vi "meas_voltmetr_with_scanner.vi"(8 "error in (no error)":errorcluster, 9 "Range":dbl=-1.0, 10 "Function":T1, 11 "output cluster in":T2) -> (0 "error out":errorcluster, 2 "value":dbl, 3 "output cluster out":T2)   [LabVIEW 2017]
uses:
  controls/app_data.ctl
  controls/instruments.ctl
  Unicorn Labview Library/Control/unicorn_Param.ctl
  Unicorn Labview Library/Control/unicorn_conn.ctl
  Unicorn Labview Library/Control/unicorn_JSON.ctl
  Unicorn Labview Library/Control/unicorn_ParamInt.ctl
  Unicorn Labview Library/Control/unicorn_Telemetry.ctl
  Unicorn Labview Library/Control/unicorn_Table.ctl
  Unicorn Labview Library/Control/unicorn_ParamFloat.ctl
  <instrlib>/PICOTEST M352XA/Public/Controls/Function.ctl
  Unicorn Labview Library/Unicorn Library.lvlib
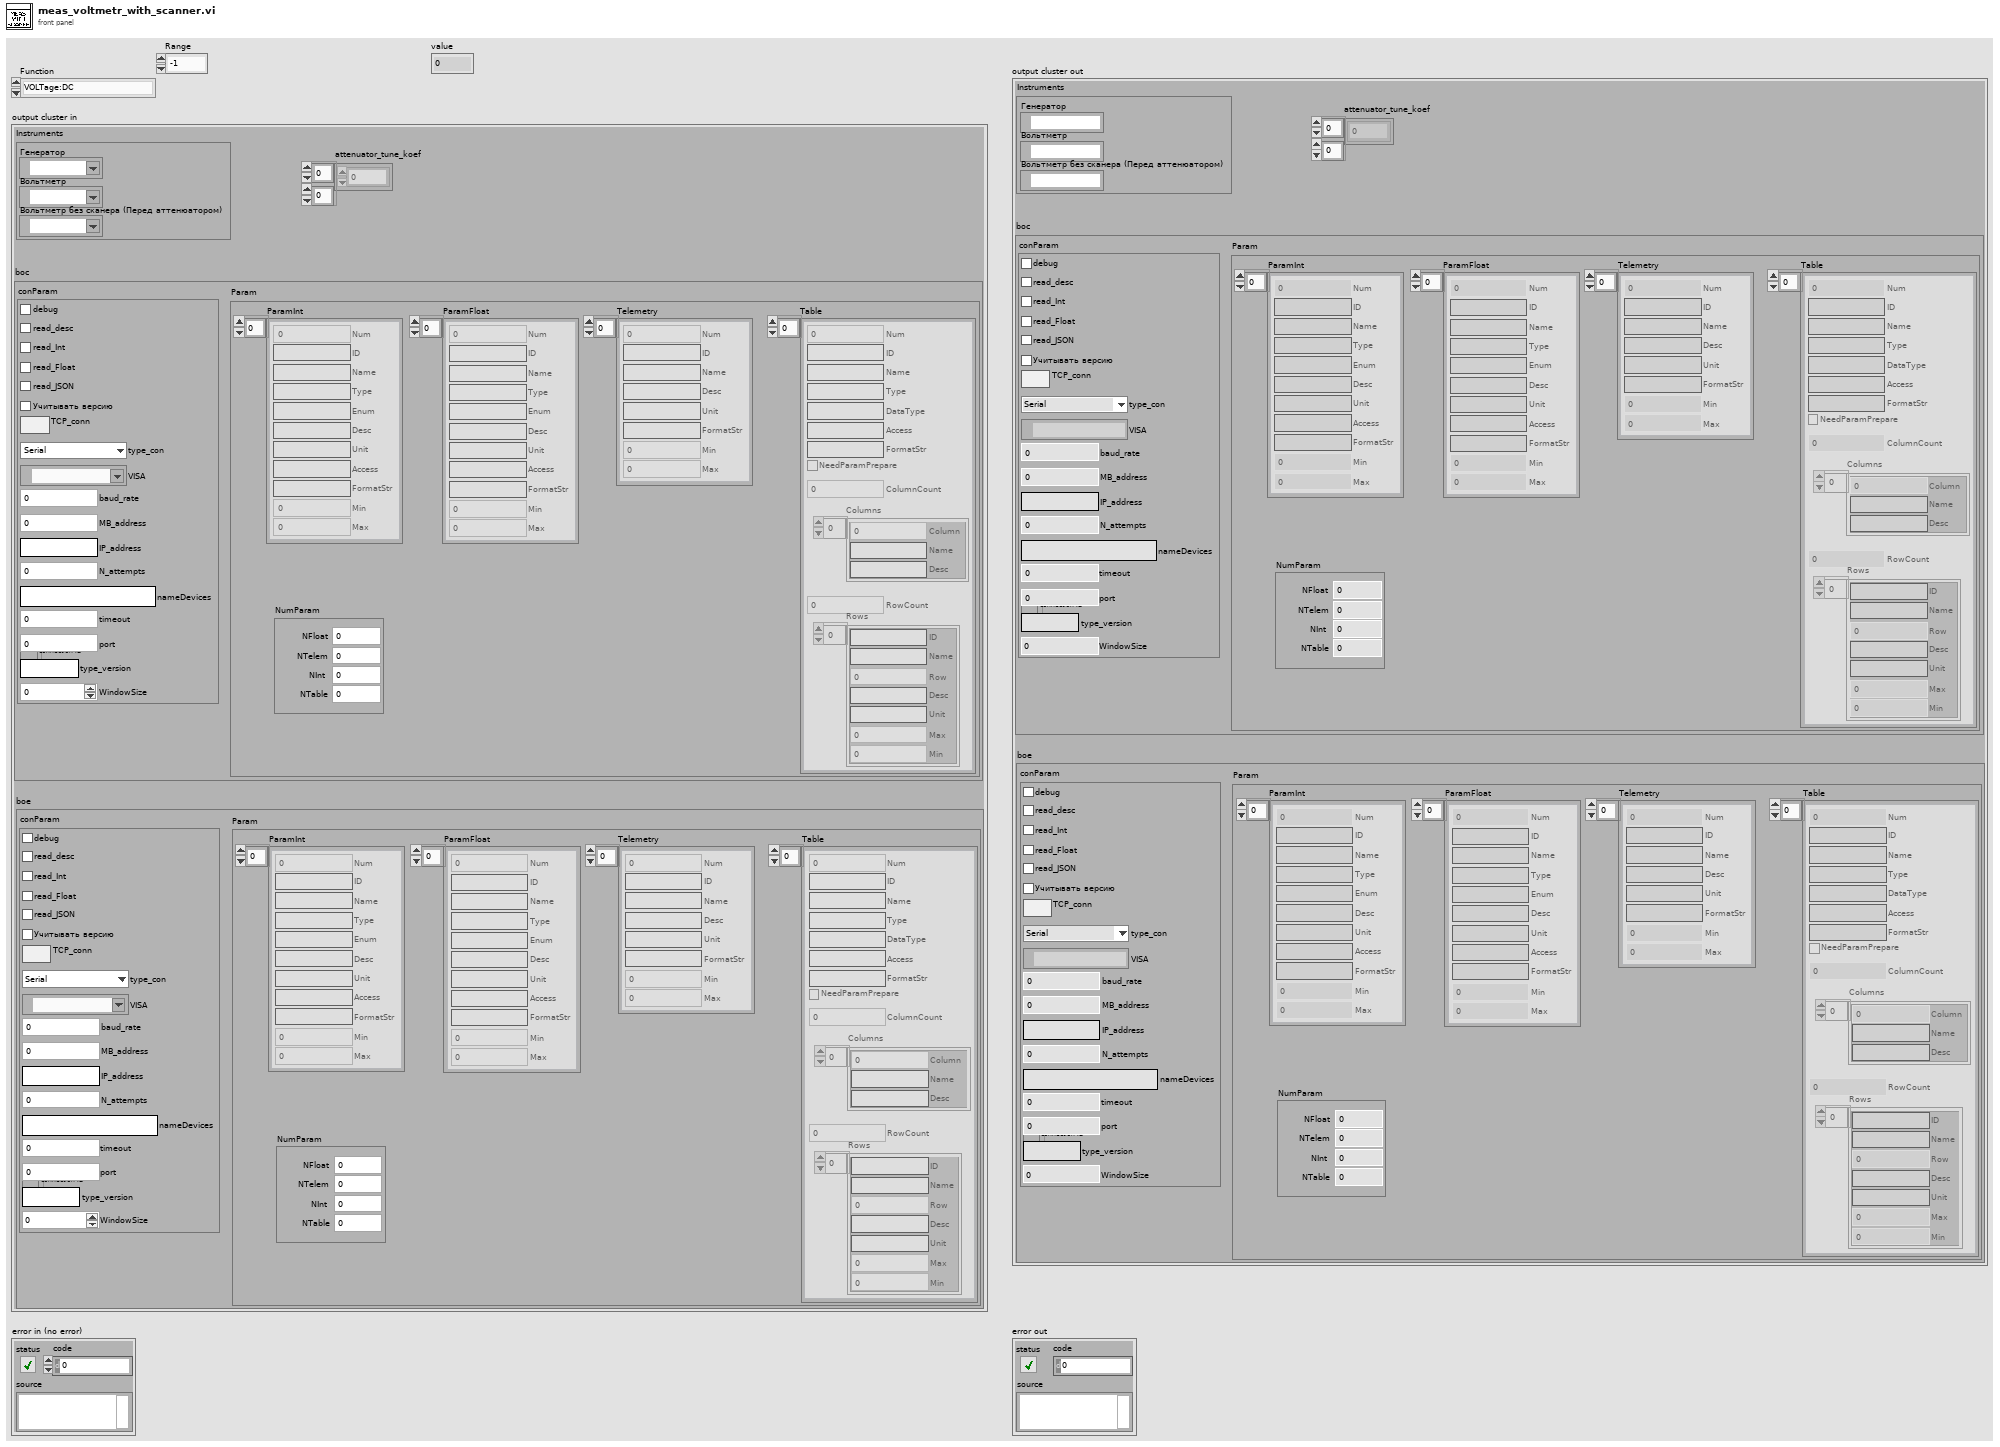
[diagram p1: front panel]
types:
  T1 = typedef "Function.ctl" = enum16{"VOLTage:DC", "VOLTage:DC:RATio", "VOLTage:AC", "CURRent:DC", "CURRent:AC", "RESistance", "FRESistance", "FREQuency", "PERiod", "FREQuency:CURRent", "PERiod:CURRent", "CAPacitance", "CONTinuity", "DIODe", "TCOuple", "TEMPerature"}
  T2 = typedef "app_data.ctl" = cluster{"Instruments":T3, "boc":T4, "boe":T4, "attenuator_tune_koef":dbl[][]}
  T3 = typedef "instruments.ctl" = cluster{"generator":refnum<visa-resource-name>, "voltment_with_scaner":refnum<visa-resource-name>, "voltment_without_scaner":refnum<visa-resource-name>}
  T4 = typedef "Unicorn Library.lvlib/unicorn_Param.ctl" = cluster{"conParam":T5, "Param":T6}
  T5 = typedef "Unicorn Library.lvlib/unicorn_conn.ctl" = cluster{"ReadIntParam":bool, "ReadDescrParam":bool, "ReadFloatParam":bool, "debug":bool, "ReadJSON":bool, "IP_address":string, "N_attempts":i32, "type_con":enum16{"Serial", "TCP"}, "MB_address":i32, "VISA":refnum<visa-resource-name>, "connection ID":refnum<k5>, "nameDevices":string, "timeout":i32, "port":u16, "type_version":string, "baud_rate":u32, "VersionControl":bool, "TCP_conn":bool, "WindowSize":i32}
  T6 = typedef "Unicorn Library.lvlib/unicorn_JSON.ctl" = cluster{"NumParam":cluster{"NTelem":i32, "NInt":i32, "NFloat":i32, "NTable":i32}, "ParamInt":T7, "Telemetry":T8, "Table":T9, "ParamFloat":T10}
  T7 = typedef "Unicorn Library.lvlib/unicorn_ParamInt.ctl" = cluster{"ID":string, "Num":i32, "Name":string, "Type":string, "Enum":string, "Desc":string, "Unit":string, "Access":string, "FormatStr":string, "Min":i32, "Max":i32}[]
  T8 = typedef "Unicorn Library.lvlib/unicorn_Telemetry.ctl" = cluster{"ID":string, "Num":i32, "Name":string, "Desc":string, "Unit":string, "FormatStr":string, "Min":i32, "Max":i32}[]
  T9 = typedef "Unicorn Library.lvlib/unicorn_Table.ctl" = cluster{"Num":i32, "Access":string, "ColumnCount":i32, "NeedParamPrepare":bool, "Columns":cluster{"Column":i32, "Desc":string, "Name":string}[], "DataType":string, "FormatStr":string, "ID":string, "Name":string, "RowCount":i32, "Rows":cluster{"Desc":string, "ID":string, "Max":i32, "Min":i32, "Name":string, "Row":i32, "Unit":string}[], "Type":string}[]
  T10 = typedef "Unicorn Library.lvlib/unicorn_ParamFloat.ctl" = cluster{"ID":string, "Num":i32, "Name":string, "Type":string, "Enum":string, "Desc":string, "Unit":string, "Access":string, "FormatStr":string, "Min":i32, "Max":i32}[]
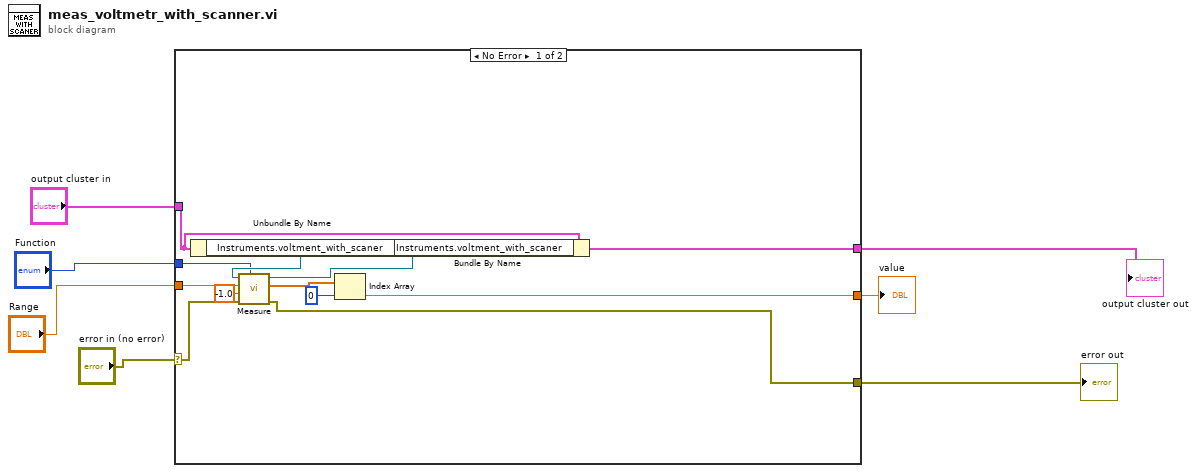
[diagram p0: block diagram]
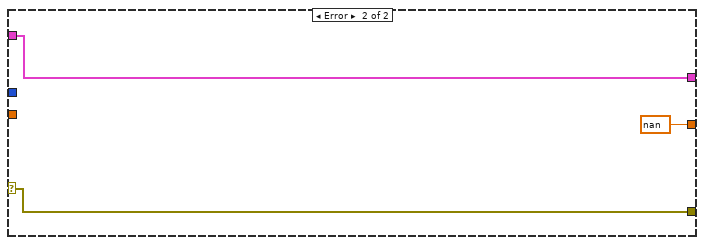
[diagram p2: hidden frame]
diagram:
  n1 = case shown="No Error" "error in (no error)" {
    selector: "error in (no error)" -> [w10 w21]
    tunnel: [w19 w22] -> w7
    tunnel: "output cluster in" -> [w18 w22]
    tunnel: [w16 w21] -> w5
    tunnel: "Function" -> [w11 _]
    tunnel: [w9 nan ("Measurement")] -> w2
    tunnel: "Range" -> [w8 _]
    frame No Error {
      n2 = Unbundle By Name(w18) -> ("Instruments.voltment_with_scaner"=w12:refnum<visa-resource-name>)
      n3 = call <instrlib>:"Measure.vi"("Function"=w11, "error in (no error)"=w10, "Resolution"=-1.0, "Range"=w8, "VISA resource name"=w12) -> ("error out"=w16:errorcluster, "Measurements"=w14:dbl[], "VISA resource name out"=w17:refnum<visa-resource-name>)  [unwired: 4 in]
      n4 = Index Array(array=w14, index=0) -> (element=w9:dbl)
      n5 = Bundle By Name(cluster=w18, "Instruments.voltment_with_scaner"=w17) -> (w19:T2)
    }
    frame Error {
    }
  }
  "output cluster out" <- w7
  "error out" <- w5
  "value" <- w2
